vi "Read Library Info File.vi"(8 "error in (no error)":errorcluster, 10 "Project Root":path, 11 "Library Info Path":path) -> (0 "error out":errorcluster, 2 "Library Info":T1, 3 "dup Library Info Path":path)   [LabVIEW 2011]
uses:
  Type Definitions/Library Information Cluster.ctl
  <vilib>/addons/_JKI.lib/File Uncertified/_R-W Text File Support/R-W Text File Mode Enum__JKI File Uncertified.ctl
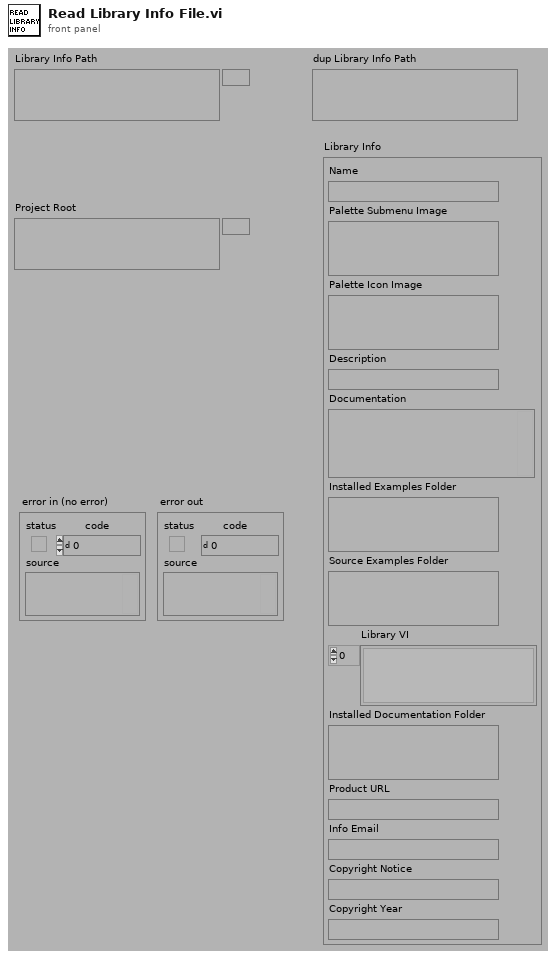
[diagram p1: front panel]
types:
  T1 = typedef "Library Information Cluster.ctl" = cluster{"Name":string, "Palette Submenu Image":path, "Palette Icon Image":path, "Description":string, "Documentation":string, "Installed Examples Folder":path, "Source Examples Folder":path, "Library VI":path[], "Installed Documentation Folder":path, "Product URL":string, "Info Email":string, "Copyright Notice":string, "Copyright Year":string}
  T2 = typedef "R-W Text File Mode Enum__JKI File Uncertified.ctl" = enum16{"read", "create", "append"}
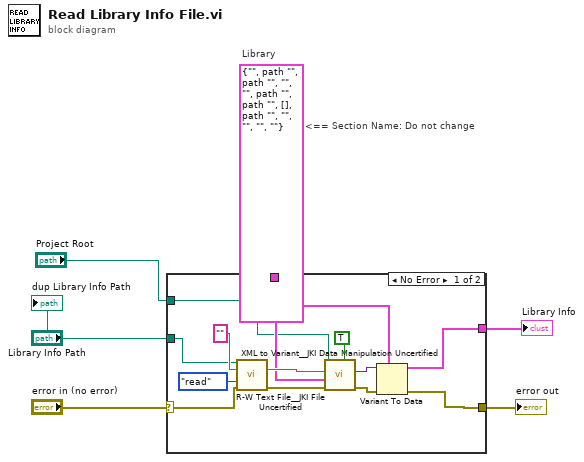
[diagram p0: block diagram]
diagram:
  w6 = T1 {"Name"="", "Palette Submenu Image"=path "", "Palette Icon Image"=path "", "Description"="", "Documentation"="", "Installed Examples Folder"=path "", "Source Examples Folder"=path "", "Library VI"=[], "Installed Documentation Folder"=path "", "Product URL"="", "Info Email"="", "Copyright Notice"="", "Copyright Year"=""}  # Library
  # "<== Section Name: Do not change"
  n1 = case shown="No Error" "error in (no error)" {
    selector: "error in (no error)" -> [w17 w20]
    tunnel: w6 -> [w14 w21]
    tunnel: [w19 w21] -> w5
    tunnel: "Library Info Path" -> [w9 _]
    tunnel: [w10 w20] -> w3
    tunnel: "Project Root" -> [w7 _]
    frame No Error {
      n2 = call <vilib>:"R-W Text File__JKI File Uncertified.vi"("Path In"=w9, "Data In"="", "Action (Read)"=R-W_Text_File_Mode_Enum__JKI_File_Uncertified."read", "error in (no error)"=w17) -> ("Data Out"=w18:string, "error out"=w13:errorcluster)  [unwired: 8 in, 2 out]
      n3 = call <vilib>:"XML to Variant__JKI Data Manipulation Uncertified.vi"("expand paths relative to \"<base>:\\\" (FALSE)"=TRUE ("expand paths relative to \"<base>:\\\" (FALSE)"), "error in (no error)"=w13, "LabVIEW Data (Type)"=w14, "XML String"=w18, "\"<base>:\\\" path (for relative)"=w7) -> ("error out"=w12:errorcluster, "LabVIEW Data"=w11:variant)  [unwired: 5 in]
      n4 = Variant To Data(error in=w12, type=w14, Variant=w11) -> (data=w19:T1, error out=w10:errorcluster)
    }
    frame Error {
    }
  }
  "Library Info" <- w5
  "error out" <- w3
  "dup Library Info Path" <- "Library Info Path"
